vi "conDisCon.vi"() -> ()   [LabVIEW 2024]
uses:
  <userlib>/er4commlib_labview/er4commlib_labview.lvlib
panel:
  out "disCon2 2":u32(ring)
  out "error out":errorcluster
  out "disCon2":u32(ring)
  in  "error in (no error)":errorcluster
  out "connectDev1":u32(ring)
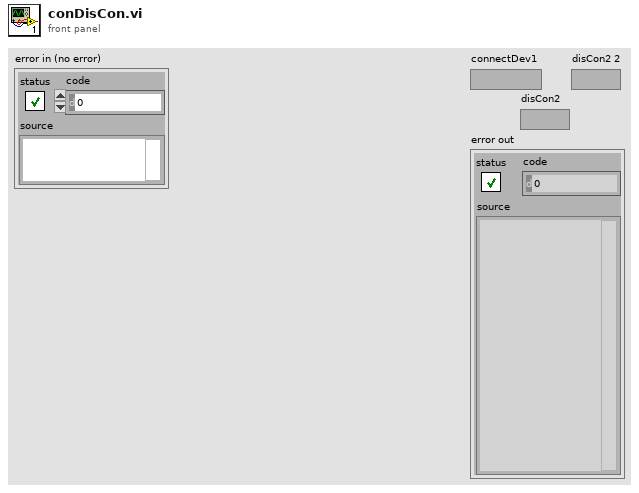
[diagram p1: front panel]
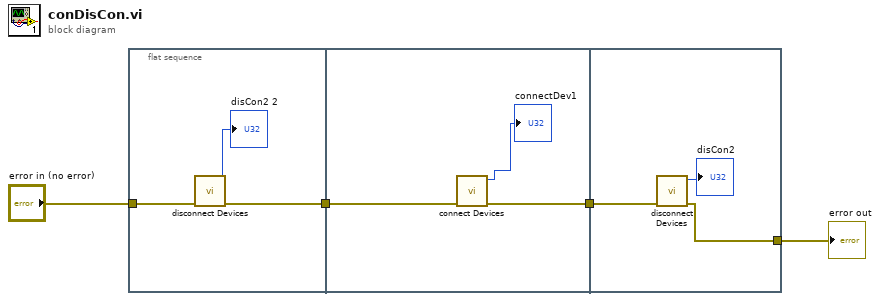
[diagram p0: block diagram]
diagram:
  n1 = flat-sequence {
    tunnel: "error in (no error)" -> [w6]
    tunnel: [w5] -> w2
    tunnel: w2 -> [w10]
    tunnel: [w8] -> w1
    tunnel: [w12] -> w3
    tunnel: w1 -> [w11]
    frame #0 {
      n2 = call <userlib>:"disconnect Devices.vi"("error in (no error)"=w6) -> ("error out"=w5:errorcluster, "function return"=→"disCon2 2":u32)  [unwired: 9 in]
    }
    frame #1 {
      n3 = call <userlib>:"connect Devices.vi"("error in (no error)"=w10) -> ("error out"=w8:errorcluster, "function return"=→"connectDev1":u32)  [unwired: 9 in]
    }
    frame #2 {
      n4 = call <userlib>:"disconnect Devices.vi"("error in (no error)"=w11) -> ("error out"=w12:errorcluster, "function return"=→"disCon2":u32)  [unwired: 9 in]
    }
  }
  "error out" <- w3
